vi "Main.vi"(8 "error in":errorcluster caption="entrée d'erreur") -> (0 "error out":errorcluster caption="sortie d'erreur")   [LabVIEW 2026]
uses:
  <instrlib>/PI/Low Level/Communication/Interface Settings.ctl
panel:
  out "Current pos (µm)":dbl
  in  "Arrêter":bool
  in  "Mov Rel (µm)":dbl
  in  "Mov Abs (µm)":dbl
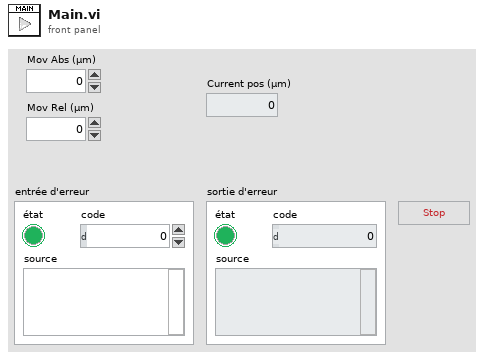
[diagram p1: front panel]
types:
  T1 = enum16{"INIT", "CLOSE", "MOVABS", "MOVREL", "POS?", "WaitForEvents"}
  T2 = typedef "Interface Settings.ctl" = cluster{"Interface":u16, "Timeout":u32, "RS232 settings":cluster{"Portnumber":u8, "Baudrate":u16}, "TCP/IP settings":cluster{"Host address/name":string, "Port":i32, "Board":i32, "TCP/IP Search?":bool}, "USB settings":cluster{"S/N":string, "USB Search?":bool}, "DaisyChain settings":cluster{"Register DC":bool, "DaisyChain Search?":bool, "Device ID":i32}, "DLL for Device":u16}
  T3 = enum16{"Do not reference", "Reference switch", "Negative limit switch", "Positive limit switch"}[]
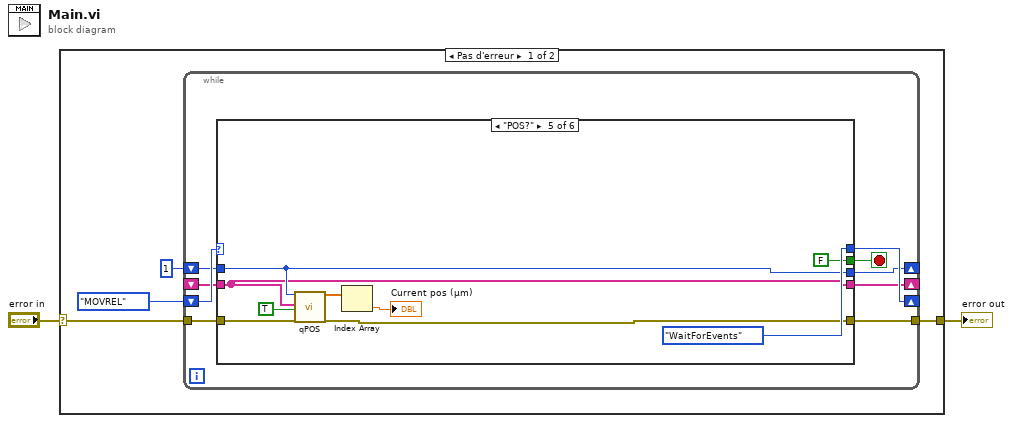
[diagram p0: block diagram]
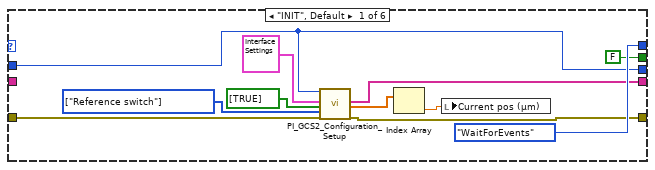
[diagram p2: hidden frame]
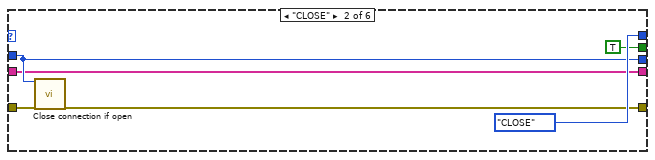
[diagram p3: hidden frame]
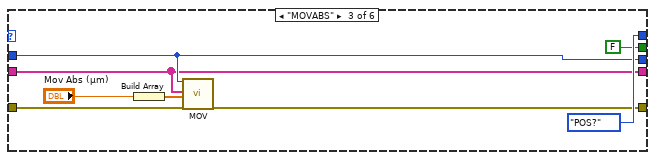
[diagram p4: hidden frame]
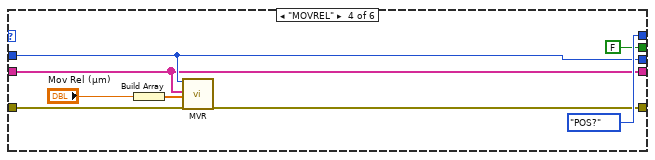
[diagram p5: hidden frame]
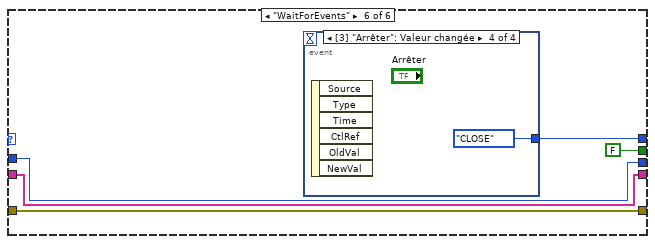
[diagram p6: hidden frame]
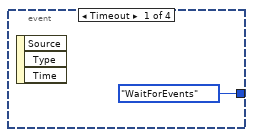
[diagram p7: hidden frame]
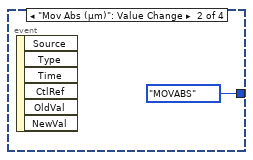
[diagram p8: hidden frame]
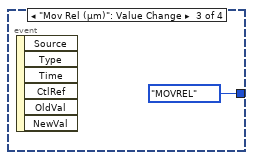
[diagram p9: hidden frame]
diagram:
  n1 = case shown="Pas d'erreur" "error in" {
    selector: "error in" -> [w5 w67]
    tunnel: [w4 w67] -> w1
    frame No Error {
      n2 = while {
        shift-right: [w14] -> _
        shift-left: T1."MOVREL" ("States") -> [w15]
        tunnel: w5 -> [w12]
        tunnel: [w11] -> w4
        shift-right: [w9] -> _
        shift-left: 1 ("System no.") -> [w10]
        shift-right: [w8] -> _
        shift-left: _ -> [w7]
        stop <- w13 stop-if-true
        n3 = case shown="\"POS?\"" w15 {
          tunnel: [T1."WaitForEvents" ("States") T1."CLOSE" ("States") T1."POS?" ("States") T1."POS?" ("States") T1."WaitForEvents" ("States") w62] -> w14
          tunnel: [FALSE TRUE FALSE FALSE FALSE FALSE] -> w13
          tunnel: w12 -> [w24 w30 w37 w46 w51 w60]
          tunnel: [w23 w29 w36 w42 w50 w60] -> w11
          tunnel: w10 -> [w17 w28 w38 w45 w55 w59]
          tunnel: [w17 w28 w38 w45 w55 w59] -> w9
          tunnel: [w16 w27 w33 w41 w49 w58] -> w8
          tunnel: w7 -> [_ w27 w33 w41 w49 w58]
          frame "INIT", Default {
            w21 = T3 [enum."Reference switch"] items=["Do not reference", "Reference switch", "Negative limit switch", "Positive limit switch"] ("Reference mode")
            n4 = call <instrlib>:"PI_GCS2_Configuration_Setup.vi"("System no."=w17, "Interface settings"=T2 {"Interface"=2, "Timeout"=5000, "RS232 settings"={"Portnumber"=1, "Baudrate"=5}, "TCP/IP settings"={"Host address/name"="localhost", "Port"=50000, "Board"=0, "TCP/IP Search?"=TRUE}, "USB settings"={"S/N"="", "USB Search?"=TRUE}, "DaisyChain settings"={"Register DC"=FALSE, "DaisyChain Search?"=TRUE, "Device ID"=1}, "DLL for Device"=17}, "Closed Loop"=bool[] [TRUE], "Reference mode"=w21, "error in"=w24) -> ("Conn. Axis"=w16:string[], "Position"=w19:dbl[], "error out"=w23:errorcluster)  [unwired: 9 in, 3 out]
            n5 = Index Array(array=w19) -> (element=w18:dbl)  [unwired: 1 in]
            n6 = local write "Current pos (µm)"(w18) -> ()
          }
          frame "CLOSE" {
            n7 = call <instrlib>:"Close connection if open.vi"("System no."=w28, "error in"=w30) -> ("error out"=w29:errorcluster)  [unwired: 16 in, 1 out]
          }
          frame "MOVABS" {
            n8 = Build Array("Mov Abs (µm)") -> (w34:dbl[])
            n9 = call <instrlib>:"MOV.vi"("System no."=w38, "Axes to move"=w33, "Position values"=w34, "error in"=w37) -> ("error out"=w36:errorcluster)  [unwired: 15 in]
          }
          frame "MOVREL" {
            n10 = Build Array("Mov Rel (µm)") -> (w43:dbl[])
            n11 = call <instrlib>:"MVR.vi"("System no."=w45, "Axes to move"=w41, "Position values"=w43, "error in"=w46) -> ("error out"=w42:errorcluster)  [unwired: 15 in]
          }
          frame "POS?" {
            n12 = call <instrlib>:"qPOS.vi"("System no."=w55, "Axes to query"=w49, "All axes?"=TRUE, "error in"=w51) -> ("Position"=w54:dbl[], "error out"=w50:errorcluster)  [unwired: 14 in]
            n13 = Index Array(array=w54) -> (element=→"Current pos (µm)":dbl)  [unwired: 1 in]
          }
          frame "WaitForEvents" {
            n14 = event shown="[3] \"Arrêter\": Valeur changée" {
              selector: _ -> [_ _ _ _]
              dyn-events: _ -> [_ _ _ _]
              timeout: _ -> [_ _ _ _]
              tunnel: [T1."WaitForEvents" ("States") T1."MOVABS" ("States") T1."MOVREL" ("States") T1."CLOSE" ("States")] -> w62
              event Timeout {
                n15 = event-data() -> ()  [unwired: 1 in, 3 out]
              }
              event "Mov Abs (µm)": Value Change {
                n16 = event-data() -> ()  [unwired: 1 in, 6 out]
              }
              event "Mov Rel (µm)": Value Change {
                n17 = event-data() -> ()  [unwired: 1 in, 6 out]
              }
              event "Arrêter": Value Change {
                n18 = event-data() -> ()  [unwired: 1 in, 6 out]
              }
            }
          }
        }
      }
    }
    frame Error {
    }
  }
  "error out" <- w1
